vi "AerotechHome.vi"(8 "error in (no error)":errorcluster) -> (0 "error out":errorcluster)   [LabVIEW 2009]
uses:
  Controls/AerotechCommand.ctl
  Controls/AerotechState.ctl
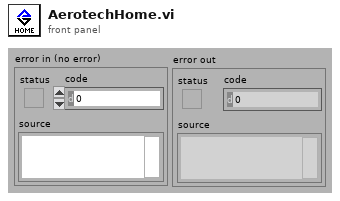
[diagram p1: front panel]
types:
  T1 = typedef "AerotechState.ctl" = enum16{"INITING", "IDLING", "SLEWING", "TRACKING", "MOVING", "HOMING", "STOPPING"}
  T2 = typedef "AerotechCommand.ctl" = enum16{"TRACK", "POSITION", "STOP", "HOME", "QUIT"}
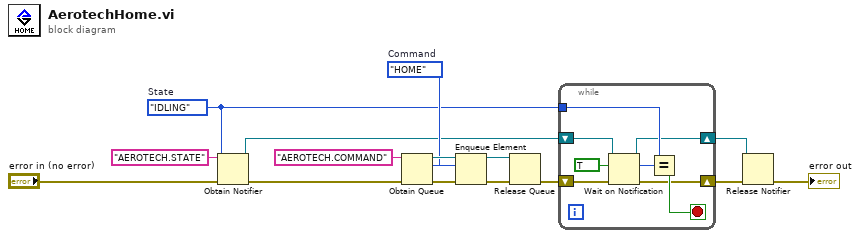
[diagram p0: block diagram]
diagram:
  w6 = AerotechState."IDLING"  # State
  w12 = AerotechCommand."HOME"  # Command
  n1 = Obtain Notifier(name (unnamed)="AEROTECH.STATE", notification data type=w6, error in (no error)="error in (no error)") -> (notifier out=w2:refnum<notifier>, error out=w1:errorcluster)  [unwired: 1 in, 1 out]
  n2 = Obtain Queue(name (unnamed)="AEROTECH.COMMAND", element data type=w12, error in (no error)=w1) -> (queue out=w13:refnum<queue>, error out=w14:errorcluster)  [unwired: 2 in, 1 out]
  n3 = Enqueue Element(queue=w13, element=w12, error in (no error)=w14) -> (queue out=w8:refnum<queue>, error out=w9:errorcluster)  [unwired: 1 in, 1 out]
  n4 = Release Queue(queue=w8, error in (no error)=w9) -> (error out=w7:errorcluster)  [unwired: 1 in, 2 out]
  n5 = while {
    shift-right: [w18] -> w5
    shift-left: w7 -> [w23]
    shift-right: [w17] -> w4
    shift-left: w2 -> [w22]
    tunnel: w6 -> [w20]
    stop <- w19 stop-if-true
    n6 = Wait on Notification(notifier=w22, ignore previous (F)=TRUE, error in (no error)=w23) -> (notifier out=w17:refnum<notifier>, notification=w21:T1, error out=w18:errorcluster)  [unwired: 1 in, 1 out]
    n7 = Equal?(x=w20, y=w21) -> (x = y?=w19:bool)
  }
  n8 = Release Notifier(notifier=w4, error in (no error)=w5) -> (error out=→"error out":errorcluster)  [unwired: 1 in, 2 out]
